vi "Update Fields Table for Spartan 5.2.vi"(8 "error in (no error)":errorcluster, 11 "Connection Refnum":T1) -> (0 "error out":errorcluster, 3 "Connection Refnum":T1)   [LabVIEW 2011]
uses:
  SI.LIB/ODBC/SQL Controls/Connection Refnum.ctl
  Field Record.ctl
  Field DataTypes.ctl
  Field NextItem.ctl
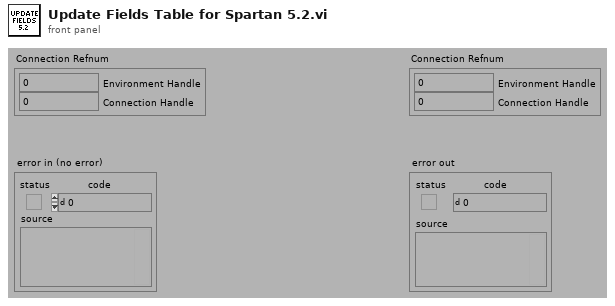
[diagram p1: front panel]
types:
  T1 = typedef "Connection Refnum.ctl" = cluster{"Environment Handle":i32, "Connection Handle":i32}
  T2 = typedef "Field Record.ctl" = cluster{"ixField":i32, "iSequenceOrder":i32, "sxFieldId":string, "sxSequenceId":string, "sDisplayName":string, "sValue":string, "sUnits":string, "nDataType":T3, "nNextItem":T4, "fSystem":bool, "fSystemValue":bool, "fRequired":bool, "fSetAtTest":bool, "fTestField":bool, "fDeleted":bool, "fIndexed":bool, "fFreeList":bool}
  T3 = typedef "Field DataTypes.ctl" = enum32{"text", "numeric", "list", "timestamp", "boolean"}
  T4 = typedef "Field NextItem.ctl" = enum32{"Reset", "Retain", "Auto-Increment"}
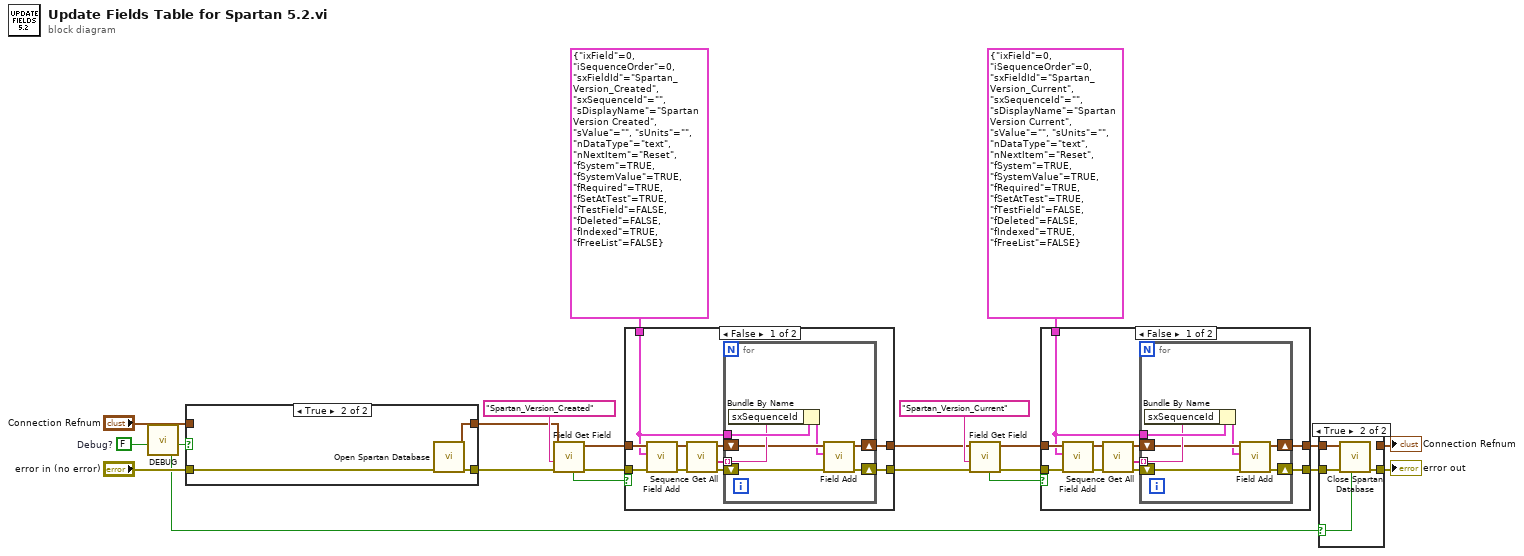
[diagram p0: block diagram]
diagram:
  w19 = FALSE  # Debug?
  n1 = call "DEBUG.vi"("Dev DEBUG? (f)"=w19) -> ("DEBUG?"=w17:bool)  [unwired: 1 in, 5 out]
  n2 = case shown="True" w17 {
    tunnel: "Connection Refnum" -> [w24 _]
    tunnel: "error in (no error)" -> [w23 w27]
    tunnel: [w23 w26] -> w14
    tunnel: [w24 w25] -> w11
    frame False {
    }
    frame True {
      n3 = call "Open Spartan Database.vi"("error in (no error)"=w27) -> ("error out"=w26:errorcluster, "Connection Refnum"=w25:T1)  [unwired: 2 in, 7 out]
    }
  }
  n4 = call "Field Get Field.vi"("error in (no error)"=w14, "sFieldId or sDisplayName (\"\")"="Spartan_Version_Created" ("sFieldId or sDisplayName (\"\")"), "Connection Refnum"=w11) -> ("error out"=w15:errorcluster, "Connection Refnum"=w12:T1, "Data Present?"=w10:bool)  [unwired: 5 in, 1 out]
  n5 = case shown="False" w10 {
    tunnel: [w28 w46] -> w3
    tunnel: [w29 w45] -> w4
    tunnel: T2 {"ixField"=0, "iSequenceOrder"=0, "sxFieldId"="Spartan_Version_Created", "sxSequenceId"="", "sDisplayName"="Spartan Version Created", "sValue"="", "sUnits"="", "nDataType"=enum."text", "nNextItem"=enum."Reset", "fSystem"=TRUE, "fSystemValue"=TRUE, "fRequired"=TRUE, "fSetAtTest"=TRUE, "fTestField"=FALSE, "fDeleted"=FALSE, "fIndexed"=TRUE, "fFreeList"=FALSE} ("Field Record") -> [w30 _]
    tunnel: w15 -> [w37 w46]
    tunnel: w12 -> [w36 w45]
    frame False {
      n6 = call "Field Add.vi"("error in (no error)"=w37, "Field Record"=w30, "Connection Refnum"=w36) -> ("error out"=w35:errorcluster, "Connection Refnum"=w34:T1)  [unwired: 6 in, 1 out]
      n7 = call "Sequence Get All.vi"("error in (no error)"=w35, "Connection Refnum"=w34) -> ("error out"=w33:errorcluster, "Sequence IDs"=w31:string[], "Connection Refnum"=w32:T1)  [unwired: 5 in, 2 out]
      n8 = for {
        shift-right: [w41] -> w29
        shift-left: w32 -> [w42]
        shift-right: [w40] -> w28
        shift-left: w33 -> [w39]
        tunnel: w31 -> [w43] mode=indexing
        tunnel: w30 -> [w44]
        n9 = Bundle By Name(cluster=w44, "sxSequenceId"=w43) -> (w38:T2)
        n10 = call "Field Add.vi"("error in (no error)"=w39, "Field Record"=w38, "Connection Refnum"=w42) -> ("error out"=w40:errorcluster, "Connection Refnum"=w41:T1)  [unwired: 6 in, 1 out]
      }
    }
    frame True {
    }
  }
  n11 = call "Field Get Field.vi"("error in (no error)"=w3, "sFieldId or sDisplayName (\"\")"="Spartan_Version_Current" ("sFieldId or sDisplayName (\"\")"), "Connection Refnum"=w4) -> ("error out"=w6:errorcluster, "Connection Refnum"=w8:T1, "Data Present?"=w9:bool)  [unwired: 5 in, 1 out]
  n12 = case shown="False" w9 {
    tunnel: [w47 w65] -> w1
    tunnel: [w48 w64] -> w2
    tunnel: T2 {"ixField"=0, "iSequenceOrder"=0, "sxFieldId"="Spartan_Version_Current", "sxSequenceId"="", "sDisplayName"="Spartan Version Current", "sValue"="", "sUnits"="", "nDataType"=enum."text", "nNextItem"=enum."Reset", "fSystem"=TRUE, "fSystemValue"=TRUE, "fRequired"=TRUE, "fSetAtTest"=TRUE, "fTestField"=FALSE, "fDeleted"=FALSE, "fIndexed"=TRUE, "fFreeList"=FALSE} ("Field Record") -> [w49 _]
    tunnel: w6 -> [w56 w65]
    tunnel: w8 -> [w55 w64]
    frame False {
      n13 = call "Field Add.vi"("error in (no error)"=w56, "Field Record"=w49, "Connection Refnum"=w55) -> ("error out"=w54:errorcluster, "Connection Refnum"=w53:T1)  [unwired: 6 in, 1 out]
      n14 = call "Sequence Get All.vi"("error in (no error)"=w54, "Connection Refnum"=w53) -> ("error out"=w52:errorcluster, "Sequence IDs"=w50:string[], "Connection Refnum"=w51:T1)  [unwired: 5 in, 2 out]
      n15 = for {
        shift-right: [w60] -> w48
        shift-left: w51 -> [w61]
        shift-right: [w59] -> w47
        shift-left: w52 -> [w58]
        tunnel: w50 -> [w62] mode=indexing
        tunnel: w49 -> [w63]
        n16 = Bundle By Name(cluster=w63, "sxSequenceId"=w62) -> (w57:T2)
        n17 = call "Field Add.vi"("error in (no error)"=w58, "Field Record"=w57, "Connection Refnum"=w61) -> ("error out"=w59:errorcluster, "Connection Refnum"=w60:T1)  [unwired: 6 in, 1 out]
      }
    }
    frame True {
    }
  }
  n18 = case shown="True" w17 {
    selector: w17 -> [_ w68]
    tunnel: w1 -> [w67 w71]
    tunnel: [w66 _] -> w18
    tunnel: [w67 w70] -> w20
    tunnel: w2 -> [w66 w69]
    frame False {
    }
    frame True {
      n19 = call "Close Spartan Database.vi"("Force Close? (f)"=w68, "error in (no error)"=w71, "Connection Refnum"=w69) -> ("error out"=w70:errorcluster)  [unwired: 2 in, 6 out]
    }
  }
  "Connection Refnum" <- w18
  "error out" <- w20
